vi "_Generate Bytes for Voltage Read.vi"(10 "Single-Diff Select (Diff)":enum16{"Differential", "Single-Ended"}(ring), 11 "Channel Select (CH0)":T1(ring)) -> (3 "Write Data1":u8[](array[numeric]))   [LabVIEW 2014]
doc: "<b>-------------------------------------------------------</b>\n** Author: Derek Murray\n** Created: 22/08/2016\n** LV Version: LabVIEW 2014 Home SP1 (14.0.1f3 32-bit)\n<b>-------------------------------------------------------</b>\n\nConfigures the bytes for MCP3008 SPI voltage read. The first byte is a write byte containing input configuration and channel selection information. The next two bytes are dummy bytes for SPI read-back from the MCP3008.\n\n<b>-------------------------------------------------------</b>\n** Copyright/License\nPermission is hereby granted, free of charge, to any person obtaining a copy of this software and associated documentation files (the \"Software\"), to deal in the Software without restriction, including without limitation the rights to use, copy, modify, merge, publish, distribute, sublicense, and/or sell copies of the Software, and to permit persons to whom the Software is furnished to do so, subject to the following conditions:\nThe above copyright notice and this permission notice shall be included in all copies or substantial portions of the Software.\nTHE SOFTWARE IS PROVIDED \"AS IS\", WITHOUT WARRANTY OF ANY KIND, EXPRESS OR IMPLIED, INCLUDING BUT NOT LIMITED TO THE WARRANTIES OF MERCHANTABILITY, FITNESS FOR A PARTICULAR PURPOSE AND NONINFRINGEMENT. IN NO EVENT SHALL THE AUTHORS OR COPYRIGHT HOLDERS BE LIABLE FOR ANY CLAIM, DAMAGES OR OTHER LIABILITY, WHETHER IN AN ACTION OF CONTRACT, TORT OR OTHERWISE, ARISING FROM, OUT OF OR IN CONNECTION WITH THE SOFTWARE OR THE USE OR OTHER DEALINGS IN THE SOFTWARE."
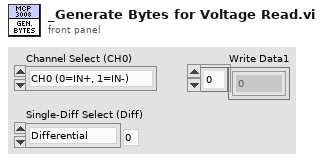
[diagram p1: front panel]
types:
  T1 = enum16{"CH0 (0=IN+, 1=IN-)", "CH1 (1=IN+, 0=IN-)", "CH2 (2=IN+, 3=IN-)", "CH3 (3=IN+, 2=IN-)", "CH4 (4=IN+, 5=IN-)", "CH5 (5=IN+, 4=IN-)", "CH6 (6=IN+, 7=IN-)", "CH7 (7=IN+, 6=IN-)"}
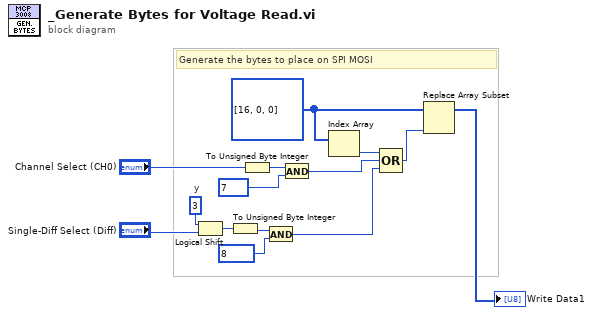
[diagram p0: block diagram]
diagram:
  w10 = u16 3  # y
  w3 = u8[] [16, 0, 0] ("Write Data1")
  # "Generate the bytes to place on SPI MOSI"
  n1 = Logical Shift(y=w10, x="Single-Diff Select (Diff)") -> (x << y=w8:u32)
  n2 = To Unsigned Byte Integer(number=w8) -> (unsigned 8bit integer=w7:u8)
  n3 = To Unsigned Byte Integer(number="Channel Select (CH0)") -> (unsigned 8bit integer=w12:u8)
  n4 = And(x=w7, y=u8 8) -> (x .and. y?=w4:u8)
  n5 = And(x=w12, y=u8 7) -> (x .and. y?=w5:u8)
  n6 = Index Array(array=w3) -> (element=w1:u8)  [unwired: 1 in]
  n7 = Compound Arithmetic op=OR(w1, w5, w4) -> (w2:u8)
  n8 = Replace Array Subset(array=w3, new element=w2) -> (→"Write Data1":u8[])  [unwired: 1 in]
